vi "Update ID.vi"(8 "error in (no error)":errorcluster, 10 "Actor ID":string, 11 "Digital Acquisition in":refnum<class "Digital Acquisition.lvclass">) -> (0 "error out":errorcluster, 3 "Digital Acquisition out":refnum<class "Digital Acquisition.lvclass">)   [LabVIEW 2020, in "Digital Acquisition.lvlib" / "Digital Acquisition.lvclass"]
uses:
  Digital Acquisition.lvclass
  Digital Acquisition.lvclass/Digital Acquisition.ctl
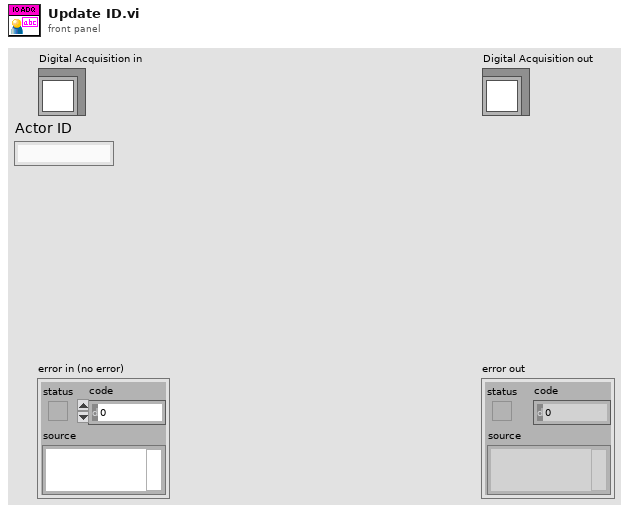
[diagram p1: front panel]
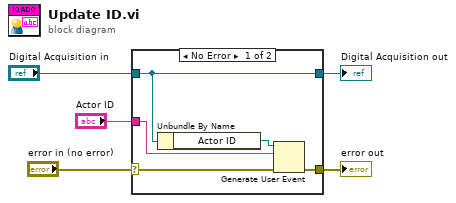
[diagram p0: block diagram]
diagram:
  n1 = case shown="No Error" "error in (no error)" {
    selector: "error in (no error)" -> [w10 w12]
    tunnel: [w9 w12] -> w4
    tunnel: [w8 w11] -> w2
    tunnel: "Digital Acquisition in" -> [w8 w11]
    tunnel: "Actor ID" -> [w6 _]
    frame No Error {
      n2 = Unbundle By Name(w8) -> ("Actor ID"=w7:refnum<user-event>)
      n3 = Generate User Event(user event=w7, event data cluster=w6, error in=w10) -> (error out=w9:errorcluster)  [unwired: 1 in, 1 out]
    }
    frame Error {
    }
  }
  "error out" <- w4
  "Digital Acquisition out" <- w2
